vi "FTW-Test-CSV-Object.vi"() -> ()   [LabVIEW 2015]
panel:
  out "CSV String":string
  out "error out":errorcluster
  in  "element":T1={"booleanfalse"=FALSE, "booleantrue"=TRUE, "U8"=8, "U16"=16, "U32"=32, "U64"=64, "I8"=-8, "I16"=-16, "I32"=-32, "I64"=-64, "SGL"=1.2345679, "DBL"=1.2345678901234567, "EXT"=1.2345678901234567, "timestamp"=timestamp(3607683703.079 s since 1904-01-01), "timestampfloat"=timestamp(3607683833 s since 1904-01-01), "stringempty"="", "stringHW"="Hello World", "EnumU8"=enum."U8", "EnumU16"=enum."U16", "EnumU32"=enum."U32", "Path"=path "c:/some folder/some file.txt", "array"=[1, 2, 3], "arrayEmpty"=[], "arrayOfClustersEmpty"=[], "visa resource"="myresource", "VIrefnum"=refnum, "subobject"={"booleanfalse"=FALSE, "booleantrue"=TRUE, "U8"=8, "U16"=16, "U32"=32, "U64"=64, "I8"=-8, "I16"=-16, "I32"=-32, "I64"=-64, "SGL"=1.2345679, "DBL"=1.2345678901234567, "EXT"=1.2345678901234567, "stringempty"="", "stringHW"="Hello World", "EnumU8"=enum."U8", "EnumU16"=enum."U16", "EnumU32"=enum."U32", "Path"=path "c:/some folder/some file.txt", "array"=[4, 5, 6], "visa resource"="myresource", "VIrefnum"=refnum}} {"timestampfloat" format="%^<%Y-%m-%dT%H:%M:%S%3uZ>T"; "timestamp" format="%^<%Y-%m-%dT%H:%M:%S%3uZ>T"; "subobject"."EXT" format="%_32g"; "subobject"."DBL" format="%_32g"; "subobject"."SGL" format="%_32g"; "EXT" format="%_32g"; "DBL" format="%_32g"; "SGL" format="%_32g"}
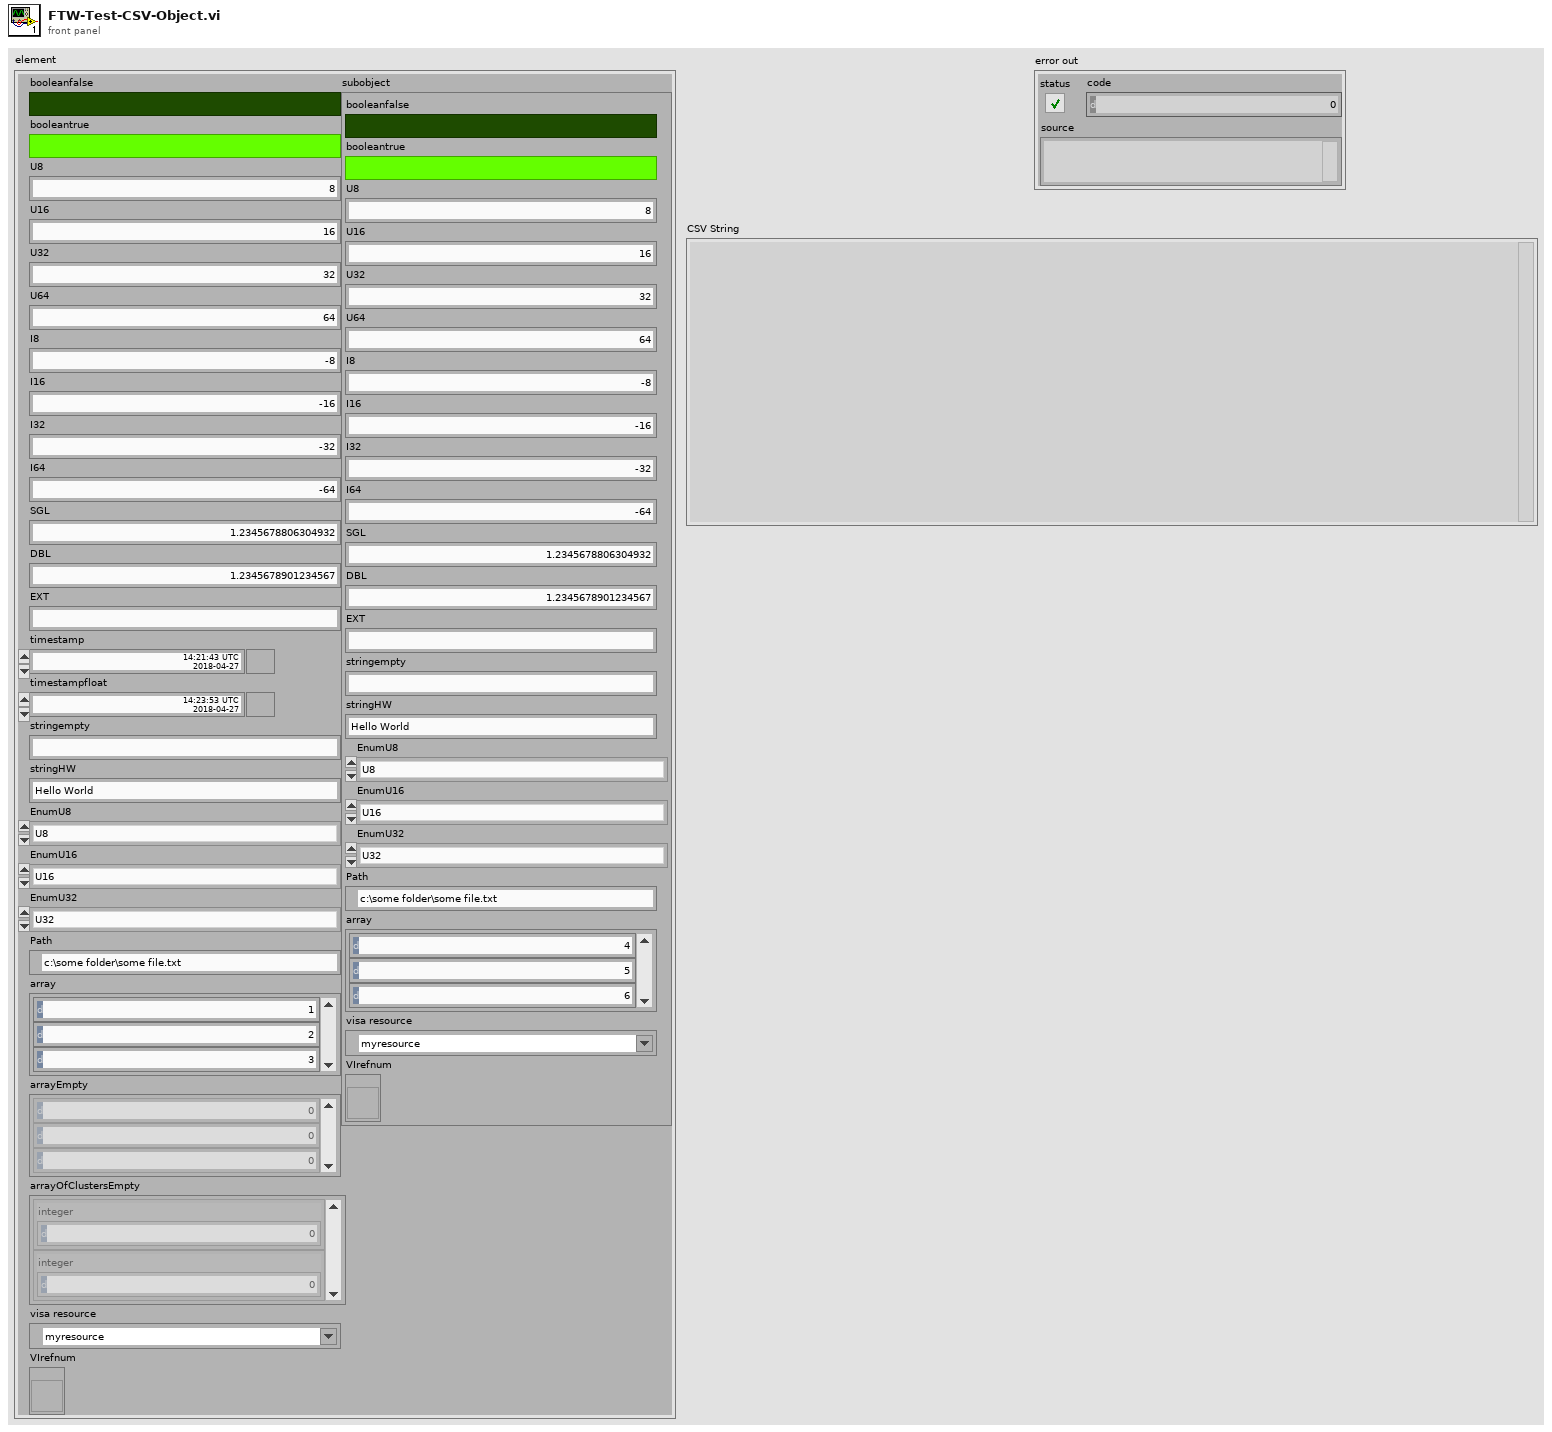
[diagram p1: front panel]
types:
  T1 = cluster{"booleanfalse":bool, "booleantrue":bool, "U8":u8, "U16":u16, "U32":u32, "U64":u64, "I8":i8, "I16":i16, "I32":i32, "I64":i64, "SGL":sgl, "DBL":dbl, "EXT":ext, "timestamp":timestamp, "timestampfloat":timestamp, "stringempty":string, "stringHW":string, "EnumU8":enum8{"unknown", "U8"}, "EnumU16":enum16{"unknown", "U16"}, "EnumU32":enum32{"unknown", "U32"}, "Path":path, "array":i32[], "arrayEmpty":i32[], "arrayOfClustersEmpty":cluster{"integer":i32}[], "visa resource":refnum<visa-resource-name>, "VIrefnum":refnum<vi>, "subobject":cluster{"booleanfalse":bool, "booleantrue":bool, "U8":u8, "U16":u16, "U32":u32, "U64":u64, "I8":i8, "I16":i16, "I32":i32, "I64":i64, "SGL":sgl, "DBL":dbl, "EXT":ext, "stringempty":string, "stringHW":string, "EnumU8":enum8{"unknown", "U8"}, "EnumU16":enum16{"unknown", "U16"}, "EnumU32":enum32{"unknown", "U32"}, "Path":path, "array":i32[], "visa resource":refnum<visa-resource-name>, "VIrefnum":refnum<vi>}}
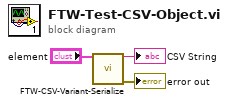
[diagram p0: block diagram]
diagram:
  n1 = call "FTW-CSV-Variant-Serialize.vi"("Variant"="element") -> ("CSV String"=→"CSV String":string, "error out"=→"error out":errorcluster)  [unwired: 13 in]
